vi "Populate Tree Control Recursive Priv.vi"(0 "Tree Dictionary In":variant, 2 "Data Types Dict":variant, 5 "TreeControl In":refnum<vi>, 7 "Child IDs":string[](array[string]), 11 "error in":errorcluster, 13 "Show IDs (True)":bool=TRUE) -> (4 "Tree Dictionary Out":variant, 6 "TreeControl Out":refnum<vi>, 15 "error out":errorcluster)   [LabVIEW 2016, in "Tree Manager.lvclass"]
uses:
  Tree Manager.lvclass
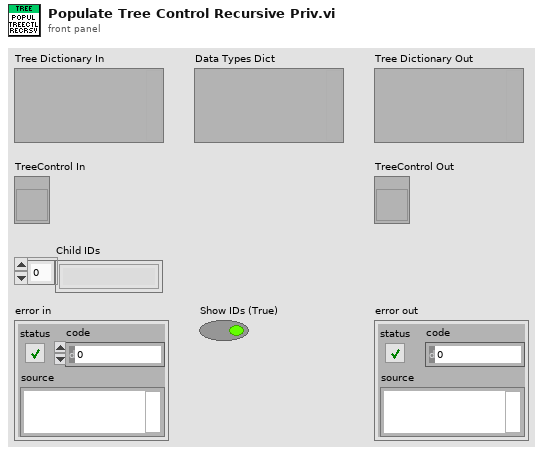
[diagram p1: front panel]
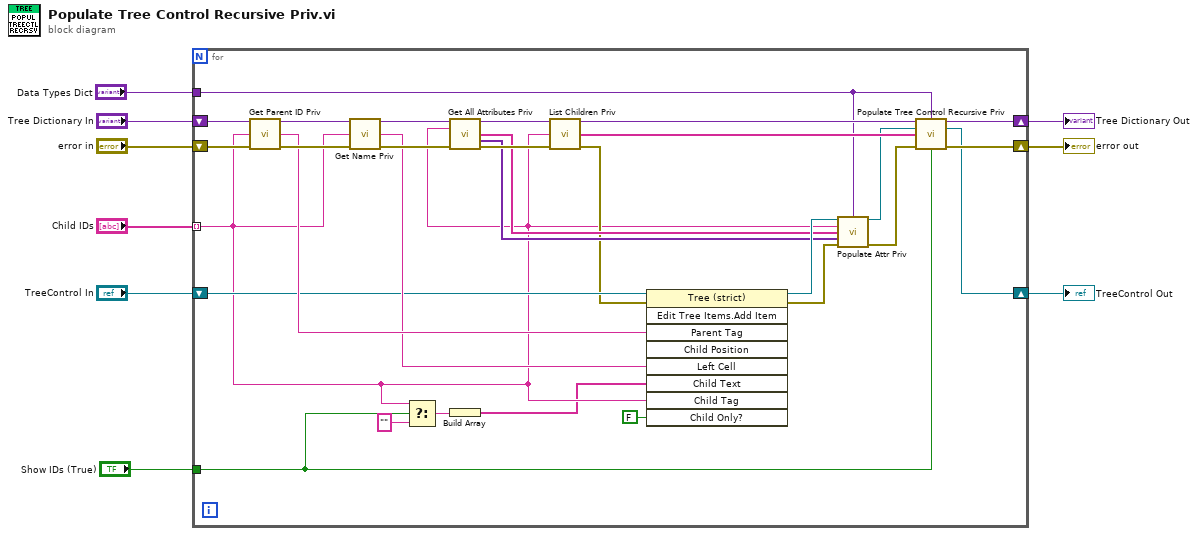
[diagram p0: block diagram]
diagram:
  n1 = for {
    tunnel: "Child IDs" -> [w15] mode=indexing
    shift-right: [w30] -> w5
    shift-left: "Tree Dictionary In" -> [w35]
    shift-right: [w28] -> w9
    shift-left: "error in" -> [w34]
    shift-right: [w26] -> w3
    shift-left: "TreeControl In" -> [w18]
    tunnel: "Show IDs (True)" -> [w14]
    tunnel: "Data Types Dict" -> [w10]
    n2 = call "Get Parent ID Priv.vi"("Tree Dictionary"=w35, "Unique ID"=w15, "error in"=w34) -> ("Tree Dictionary Out"=w33:variant, "Parent ID"=w25:string, "error out"=w32:errorcluster)  [unwired: 10 in]
    n3 = call "Get Name Priv.vi"("Tree Dictionary"=w33, "Unique ID"=w15, "error in"=w32) -> ("Tree Dictionary Out"=w39:variant, "Name"=w21:string, "error out"=w37:errorcluster)  [unwired: 10 in]
    n4 = Select(t=w15, s=w14, f="") -> (s? t:f=w12:string)
    n5 = call "Get All Attributes Priv.vi"("Tree Dictionary In"=w39, "Unique ID"=w15, "error in"=w37) -> ("Tree Dictionary Out"=w38:variant, "Attribute Names"=w20:string[], "Attribute Values"=w19:variant[], "error out"=w36:errorcluster)  [unwired: 9 in]
    n6 = Build Array(w12) -> (w11:string[])
    n7 = call "List Children Priv.vi"("Tree Dictionary"=w38, "Parent ID"=w15, "Error In"=w36) -> ("Tree Dictionary Out"=w31:variant, "Child IDs"=w29:string[], "Error Out"=w17:errorcluster)  [unwired: 10 in]
    n8 = invoke class="Tree (strict)" method="Edit Tree Items.Add Item"(reference=w18, error in=w17, "Parent Tag"=w25, "Left Cell"=w21, "Child Text"=w11, "Child Tag"=w15, "Child Only?"=FALSE) -> (reference out=w24:refnum<vi>, error out=w23:errorcluster)  [unwired: 2 in, 7 out]
    n9 = call "Populate Attr Priv.vi"("TreeControl in"=w24, "Data Types Dict"=w10, "Unique ID"=w15, "Attribute Names"=w20, "Attribute Values"=w19, "error in"=w23) -> ("TreeControl out"=w27:refnum<vi>, "error out"=w22:errorcluster)  [unwired: 8 in]
    n10 = call "Populate Tree Control Recursive Priv.vi"("Tree Dictionary In"=w31, "Data Types Dict"=w10, "TreeControl In"=w27, "Child IDs"=w29, "error in"=w22, "Show IDs (True)"=w14) -> ("Tree Dictionary Out"=w30:variant, "TreeControl Out"=w26:refnum<vi>, "error out"=w28:errorcluster)  [unwired: 7 in]
  }
  "error out" <- w9
  "Tree Dictionary Out" <- w5
  "TreeControl Out" <- w3
